vi "xString Array To XML Strings.vi"(1 "Channel On/Off":bool[](array[boolean]), 2 "index":i32, 3 "String array name":string, 4 "String array":string[](array[string])) -> (0 "xml string":string)   [LabVIEW 2012]
uses:
  xString To XML String.vi
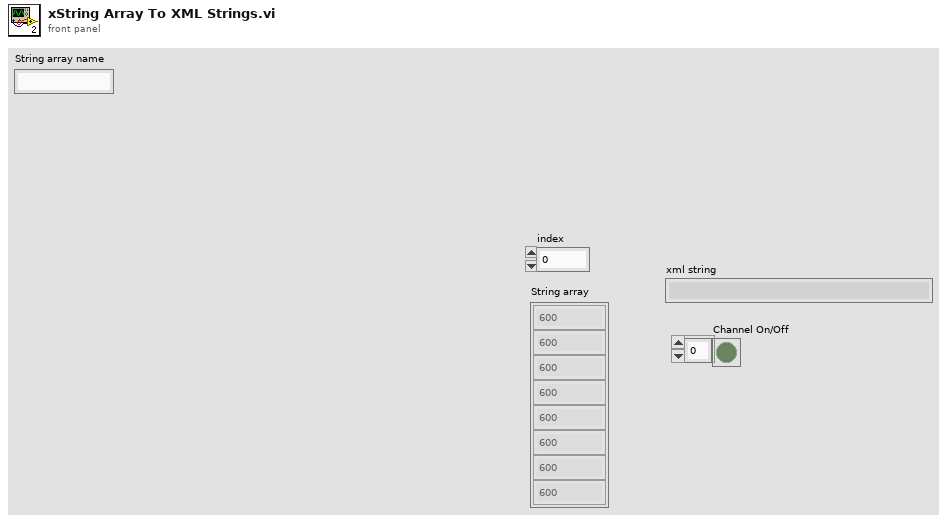
[diagram p1: front panel]
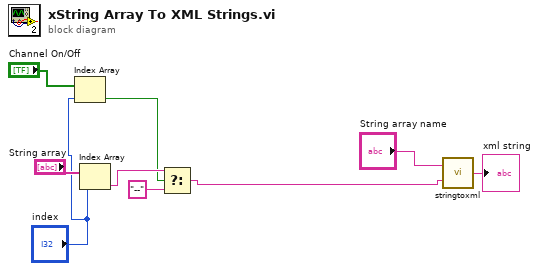
[diagram p0: block diagram]
diagram:
  n1 = Index Array(array="Channel On/Off", index="index") -> (element=w2:bool)
  n2 = Index Array(array="String array", index="index") -> (element=w8:string)
  n3 = Select(t=w8, s=w2, f="--") -> (s? t:f=w6:string)
  n4 = call "stringtoxml.vi"("String to write"=w6, "XML Tag"="String array name") -> ("xml string"=→"xml string":string)
